vi "Actor Core.vi"(8 "error in":errorcluster, 11 "Lite Tools View in":refnum<class "Lite Tools View.lvclass">) -> (0 "error out":errorcluster, 3 "Actor out":refnum<class "Actor.lvclass">)   [LabVIEW 2020, in "Lite Tools View.lvlib" / "Lite Tools View.lvclass"]
doc: "(<B>Filename</B>: Actor Framework.lvlib:Actor.lvclass:Actor Core.vi)\n\nReceives messages to the actor, reacts to them, and initiates any error handling that may shut the actor down.\n\nDescendant classes may override this VI to append parallel tasks for the actor to complete while it handles messages. Overrides use the Call Parent Method node."
uses:
  Lite Tools View.lvclass
  C:/Program Files/National Instruments/LabVIEW 2020/vi.lib/ActorFramework/Actor/Actor.lvclass
  <vilib>/ActorFramework/Actor/Actor.lvclass
  Lite Tools View.lvclass/Lite Tools View.ctl
  <vilib>/ActorFramework/Actor/Actor.lvclass/Actor.ctl
  <vilib>/ActorFramework/Message Enqueuer/Message Enqueuer.lvclass/Message Enqueuer.ctl
  Type Definitions/Tool Buttons.ctl
  Lite Tools View Messages/Broadcast Tool Buttons Pressed Msg/Broadcast Tool Buttons Pressed Msg.lvclass/Broadcast Tool Buttons Pressed Msg.ctl
  <vilib>/ActorFramework/Message Enqueuer/Init from Existing Queue.vi
  <vilib>/ActorFramework/Message Enqueuer/Enqueue.vi
  Lite Tools View Messages/Broadcast Tool Buttons Pressed Msg/Broadcast Tool Buttons Pressed Msg.lvclass
  C:/Program Files/National Instruments/LabVIEW 2020/vi.lib/ActorFramework/Message/Message.lvclass
  <vilib>/ActorFramework/Message Priority Queue/Priority Enqueue.vi
  <vilib>/ActorFrameworkMVC/Abstract View/Abstract View/Abstract View.lvclass
  <vilib>/ActorFramework/Message Enqueuer/Message Enqueuer.lvclass
panel:
  in  "Disabled Crop Button":bool
  in  "Disabled Deselect Button":bool
  in  "Tool Buttons":T1(radio)=enum."Eraser Button"
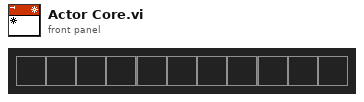
[diagram p1: front panel]
types:
  T1 = enum32{"Pan Button", "Pencil Button", "Line Button", "Eraser Button", "Rectangle Select Button", "Deselect Button", "Crop Button", "Rotate  Button", "Set Origin Button", "Zoom In Button", "Zoom Out Button"}
  T2 = enum8{"Enabled", "Disabled", "Disabled and Grayed Out"}
  T3 = typedef "Tool Buttons.ctl" = enum32{"Pan Button", "Pencil Button", "Line Button", "Eraser Button", "Rectangle Select Button", "Deselect Button", "Crop Button", "Rotate Button", "Set Origin Button", "Zoom In Button", "Zoom Out Button"}
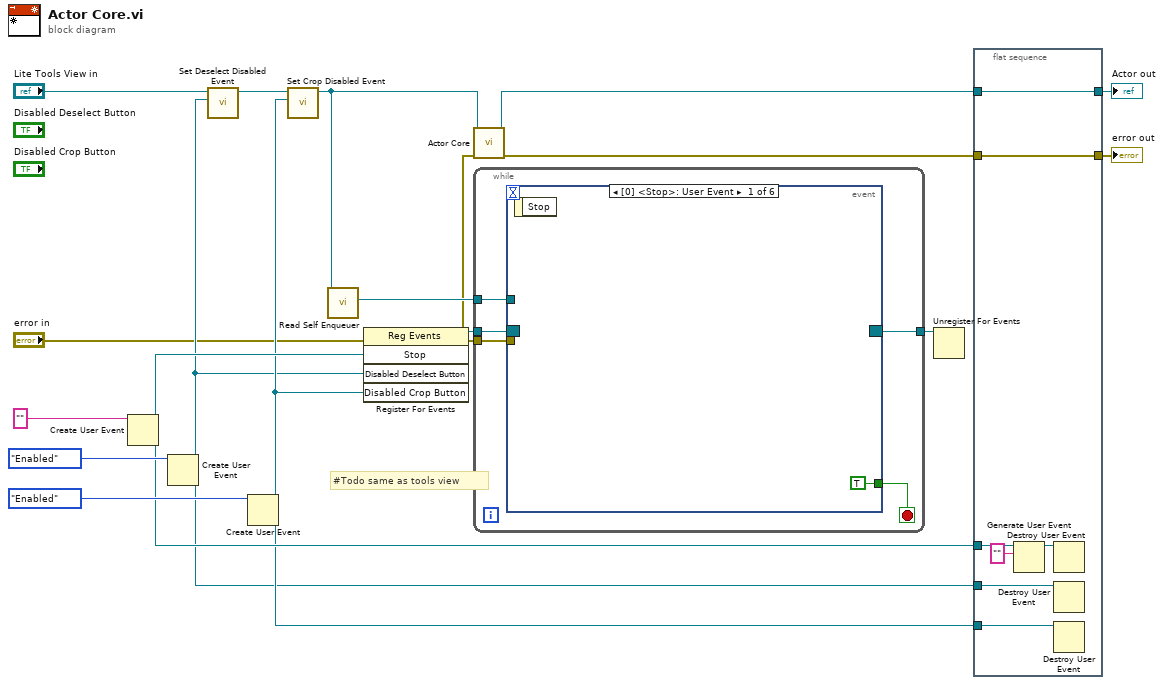
[diagram p0: block diagram]
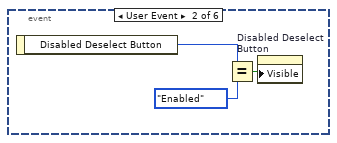
[diagram p2: hidden frame]
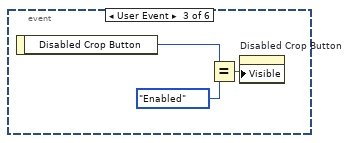
[diagram p3: hidden frame]
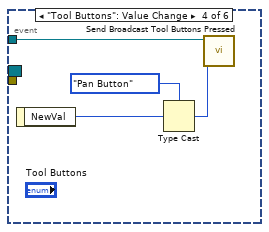
[diagram p4: hidden frame]
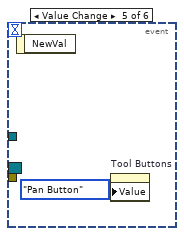
[diagram p5: hidden frame]
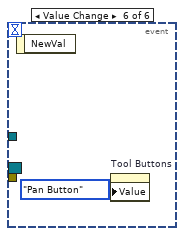
[diagram p6: hidden frame]
diagram:
  # "#Todo same as tools view"
  n1 = Create User Event(user event datatype="" ("Stop")) -> (user event=w12:refnum<user-event>)  [unwired: 1 in, 1 out]
  n2 = Create User Event(user event datatype=T2."Enabled" ("Disabled Deselect Button")) -> (user event=w7:refnum<user-event>)  [unwired: 1 in, 1 out]
  n3 = call "Set Deselect Disabled Event.vi"("Deselect Disabled Event"=w7, "Lite Tools View in"="Lite Tools View in") -> ("Lite Tools View out"=w9:refnum<class "Lite Tools View.lvclass">)  [unwired: 9 in]
  n4 = Create User Event(user event datatype=T2."Enabled" ("Disabled Crop Button")) -> (user event=w8:refnum<user-event>)  [unwired: 1 in, 1 out]
  n5 = call "Set Crop Disabled Event.vi"("Crop Disabled Event"=w8, "Lite Tools View in"=w9) -> ("Lite Tools View out"=w6:refnum<class "Lite Tools View.lvclass">)  [unwired: 9 in]
  n6 = call <vilib>:"Read Self Enqueuer.vi"("Actor"=w6) -> ("Self Enqueuer"=w13:refnum<class "Message Enqueuer.lvclass">)  [unwired: 10 in]
  n7 = register-events(error in="error in", w12, w7, w8) -> (reference out=w14:refnum<event-registration>, error out=w1:errorcluster)  [unwired: 1 in]
  n8 = call-parent "Actor Core.vi"("error in"=w1, "Abstract View in"=w6) -> ("error out"=w11:errorcluster, "Actor out"=w10:refnum<class "Actor.lvclass">)  [unwired: 8 in]
  n9 = while {
    tunnel: w14 -> [w23]
    tunnel: [w22] -> w15
    tunnel: w13 -> [w20]
    tunnel: w1 -> [w19]
    stop <- w21 stop-if-true
    n10 = event shown="[0] <Stop>: User Event" {
      selector: w23 -> [_ _ _ _ _ _]
      dyn-events: [_ _ _ _ _ _] -> w22
      timeout: _ -> [_ _ _ _ _ _]
      tunnel: [TRUE _ _ _ _ _] -> w21
      tunnel: w20 -> [_ _ _ w34 _ _]
      tunnel: w19 -> [_ _ _ _ _ _]
      event User Event {
        n11 = event-data() -> ()  [unwired: 1 in, 1 out]
      }
      event User Event {
        n12 = event-data() -> ("Disabled Deselect Button"=w27:T2)  [unwired: 1 in]
        n13 = Equal?(x=w27, y=T2."Enabled") -> (x = y?=w25:bool)
        n14 = property on="Disabled Deselect Button" class="Bool"("Visible"=w25) -> ()  [unwired: 2 in, 2 out]
      }
      event User Event {
        n15 = event-data() -> ("Disabled Crop Button"=w30:T2)  [unwired: 1 in]
        n16 = Equal?(x=w30, y=T2."Enabled") -> (x = y?=w28:bool)
        n17 = property on="Disabled Crop Button" class="Bool"("Visible"=w28) -> ()  [unwired: 2 in, 2 out]
      }
      event "Tool Buttons": Value Change {
        n18 = event-data() -> ("NewVal"=w33:T1)  [unwired: 1 in]
        n19 = Type Cast(type=Tool_Buttons."Pan Button" ("Tool Buttons"), x=w33) -> (*(type *) &x=w32:T3)
        n20 = call "Send Broadcast Tool Buttons Pressed.vi"("Tool Buttons Pressed"=w32, "Message Enqueuer"=w34) -> ()  [unwired: 8 in, 2 out]
      }
      event "Tool Buttons.Deselect Button": Value Change {
        n21 = event-data() -> ()  [unwired: 1 in, 1 out]
        n22 = property on="Tool Buttons" class="RadioBtnsControl (strict)"("Value"=T1."Pan Button" ("Tool Buttons")) -> ()  [unwired: 2 in, 2 out]
      }
      event "Tool Buttons.Crop Button": Value Change {
        n23 = event-data() -> ()  [unwired: 1 in, 1 out]
        n24 = property on="Tool Buttons" class="RadioBtnsControl (strict)"("Value"=T1."Pan Button" ("Tool Buttons")) -> ()  [unwired: 2 in, 2 out]
      }
    }
  }
  n25 = Unregister For Events(event registration refnum=w15) -> ()  [unwired: 1 in, 1 out]
  n26 = flat-sequence {
    tunnel: w12 -> [w42]
    tunnel: w7 -> [w40]
    tunnel: w8 -> [w39]
    tunnel: w10 -> [w38]
    tunnel: [w38] -> w4
    tunnel: [w37] -> w3
    tunnel: w11 -> [w37]
    frame #0 {
      n27 = Generate User Event(user event=w42, event data cluster="" ("event data")) -> (user event out=w43:refnum<user-event>)  [unwired: 2 in, 1 out]
      n28 = Destroy User Event(user event=w43) -> ()  [unwired: 1 in, 1 out]
      n29 = Destroy User Event(user event=w40) -> ()  [unwired: 1 in, 1 out]
      n30 = Destroy User Event(user event=w39) -> ()  [unwired: 1 in, 1 out]
    }
  }
  "error out" <- w3
  "Actor out" <- w4
